vi "OI global.vi"() -> ()   [LabVIEW 8.6]
panel:
  out "High Torque":bool
  out "180 turn":bool
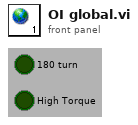
[diagram p1: front panel]
diagram:
